vi "third childs.vi"(8 "SN":string, 9 "third test item name":string, 10 "third result":string[][](array[string]), 11 "all rows":string[][](array[string]) caption="dataSource") -> (0 "thirdChilds":string)   [LabVIEW 2011]
panel:
  in  "pointSpec":string[][](array[string])
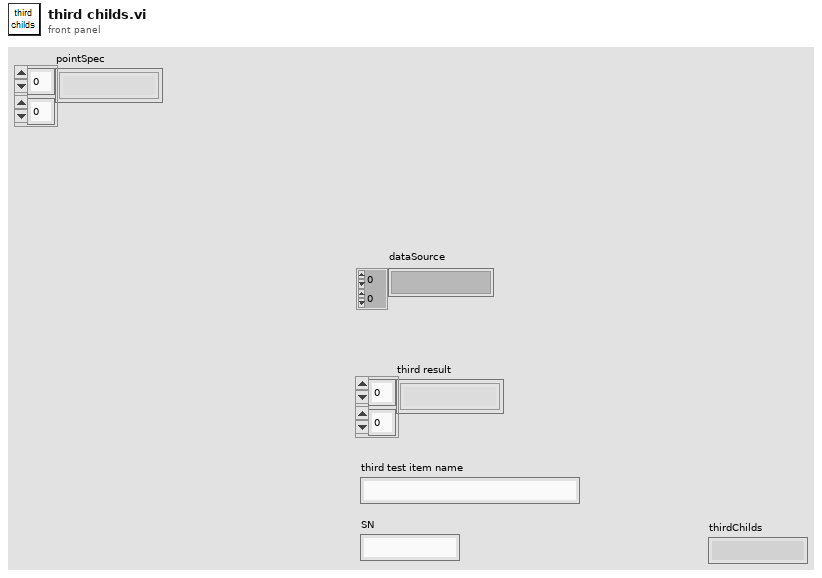
[diagram p1: front panel]
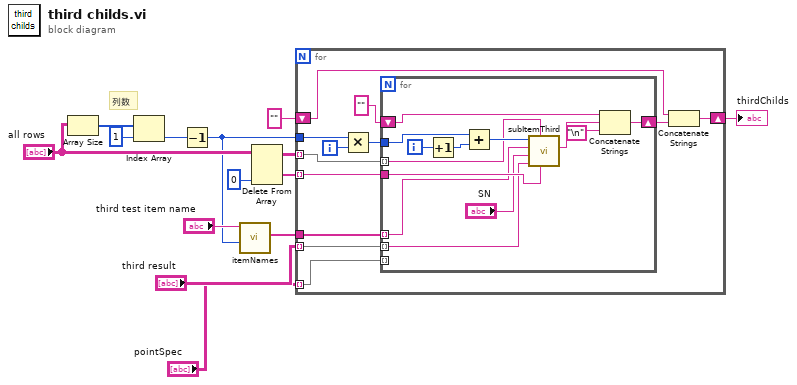
[diagram p0: block diagram]
diagram:
  # "列数"
  n1 = Array Size(array="all rows") -> (size(s)=w14:i32[])
  n2 = Index Array(array=w14, index=1 ("索引")) -> (element=w5:i32)
  n3 = Decrement(x=w5) -> (x-1=w3:i32)
  n4 = call "itemNames.vi"("pair"=w3, "itemName"="third test item name") -> ("itemNameArray"=w4:string[])  [unwired: 9 in]
  n5 = Delete From Array(array="all rows", index (col)=0 ("禁用的索引 (列)")) -> (deleted portion=w7:string[], array with subset deleted=w8:string[][])  [unwired: 2 in]
  n6 = for {
    tunnel: w3 -> [w25]
    tunnel: "third result" -> [w23] mode=indexing
    shift-right: [w19] -> w11
    shift-left: "" -> [w21]
    tunnel: w8 -> [w18] mode=indexing
    tunnel: w7 -> [w17] mode=indexing
    tunnel: w4 -> [w16]
    tunnel: "pointSpec" -> [w15] mode=indexing
    i -> [w26]
    n7 = Multiply(x=w25, y=w26) -> (x*y=w24:i32)
    n8 = for {
      tunnel: w18 -> [w36] mode=indexing
      tunnel: w24 -> [w39]
      tunnel: w17 -> [w37]
      tunnel: w23 -> [w35] mode=indexing
      shift-right: [w30] -> w20
      shift-left: "" -> [w32]
      tunnel: w16 -> [w27] mode=indexing
      tunnel: w15 -> [_] mode=indexing
      i -> [w29]
      n9 = Increment(x=w29) -> (x+1=w28:i32)
      n10 = Add(x=w39, y=w28) -> (x+y=w38:i32)
      n11 = call "subItemThird.vi"("single frequency"=w37, "single frequency value"=w36, "single frequency result"=w35, "SN"="SN", "third test item name"=w27, "subIDcount"=w38) -> ("SubItem"=w31:string)  [unwired: 5 in]
      n12 = Concatenate Strings(w32, w31, "\n") -> (w30:string)
    }
    n13 = Concatenate Strings(w21, w20) -> (w19:string)
  }
  "thirdChilds" <- w11
